vi "controlRealtimeInputLoopMode.vi"(7 "Set":bool, 8 "error in":errorcluster, 9 "RT Loop in":i32, 10 "axis in":u8, 11 "connection ID":refnum<k5>) -> (0 "error out":errorcluster, 1 "RT Loop out":i32, 2 "axis out":u8, 3 "connection ID":refnum<k5>)   [LabVIEW 2016]
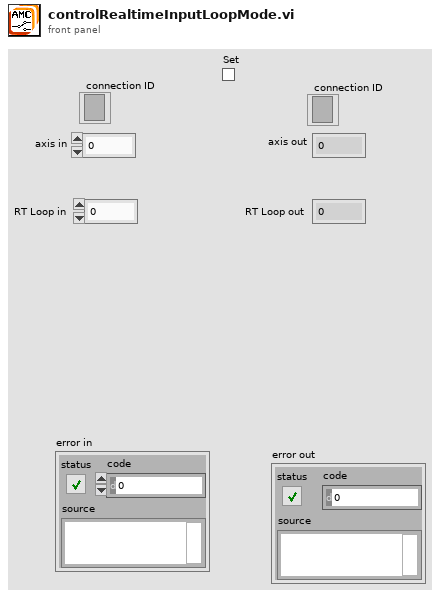
[diagram p1: front panel]
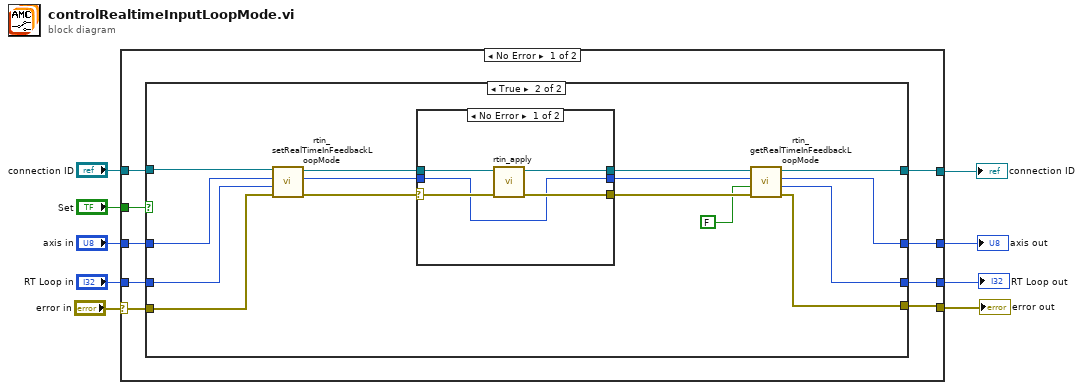
[diagram p0: block diagram]
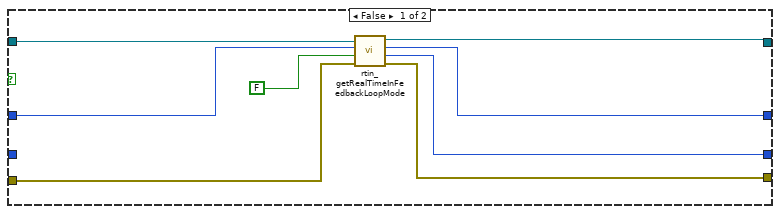
[diagram p2: hidden frame]
diagram:
  n1 = case shown="No Error" "error in" {
    selector: "error in" -> [w12 w53]
    tunnel: "axis in" -> [w16 w51]
    tunnel: [w13 w53] -> w8
    tunnel: [w11 w51] -> w7
    tunnel: "Set" -> [w17 _]
    tunnel: [w14 w50] -> w5
    tunnel: "connection ID" -> [w18 w50]
    tunnel: "RT Loop in" -> [w15 w52]
    tunnel: [w10 w52] -> w2
    frame No Error {
      n2 = case shown="True" w17 {
        tunnel: [w25 w33] -> w14
        tunnel: w18 -> [w26 w41]
        tunnel: w16 -> [w22 w39]
        tunnel: [w23 w31] -> w13
        tunnel: w15 -> [_ w37]
        tunnel: w12 -> [w24 w36]
        tunnel: [w21 w29] -> w11
        tunnel: [w20 w30] -> w10
        frame False {
          n3 = call "rtin_getRealTimeInFeedbackLoopMode.vi"("error in"=w24, "tempvalue"=FALSE, "axis"=w22, "connection ID"=w26) -> ("error out"=w23:errorcluster, "mode"=w20:i32, "axis_out"=w21:i32, "connection ID"=w25:refnum<k5>)  [unwired: 4 in]
        }
        frame True {
          n4 = call "rtin_setRealTimeInFeedbackLoopMode.vi"("error in"=w36, "mode"=w37, "axis"=w39, "connection ID"=w41) -> ("error out"=w35:errorcluster, "axis_out"=w38:i32, "connection ID"=w40:refnum<k5>)  [unwired: 5 in]
          n5 = case shown="No Error" w35 {
            selector: w35 -> [w44 w49]
            tunnel: [w43 w49] -> w32
            tunnel: w40 -> [w46 w48]
            tunnel: [w45 w48] -> w34
            tunnel: w38 -> [w42 w47]
            tunnel: [w42 w47] -> w28
            frame No Error {
              n6 = call "rtin_apply.vi"("error in"=w44, "connection ID"=w46) -> ("error out"=w43:errorcluster, "connection ID"=w45:refnum<k5>)  [unwired: 8 in]
            }
            frame Error {
            }
          }
          n7 = call "rtin_getRealTimeInFeedbackLoopMode.vi"("error in"=w32, "tempvalue"=FALSE, "axis"=w28, "connection ID"=w34) -> ("error out"=w31:errorcluster, "mode"=w30:i32, "axis_out"=w29:i32, "connection ID"=w33:refnum<k5>)  [unwired: 4 in]
        }
      }
    }
    frame Error {
    }
  }
  "error out" <- w8
  "axis out" <- w7
  "connection ID" <- w5
  "RT Loop out" <- w2
